vi "fgv_loop-dt_values.vi"() -> ()   [LabVIEW 2018]
panel:
  out "dt time arrays out":T1
  in  "dt time arrays":T1
  in  "cmd":enum16{"write", "read"}(ring)
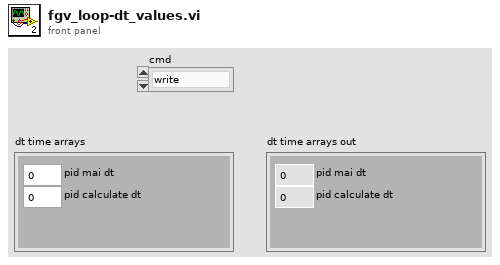
[diagram p1: front panel]
types:
  T1 = cluster{"pid mai dt":dbl, "pid calculate dt":dbl}
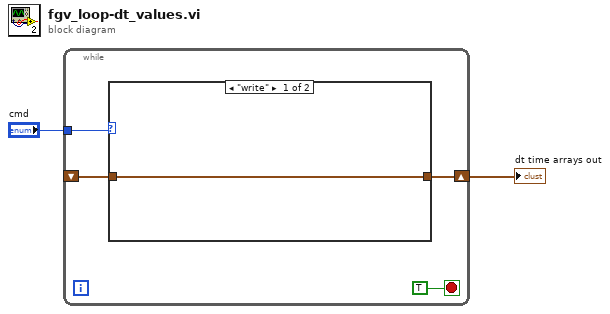
[diagram p0: block diagram]
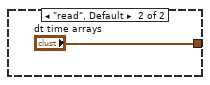
[diagram p2: hidden frame]
diagram:
  n1 = while {
    tunnel: "cmd" -> [w6]
    shift-right: [w4] -> w1
    shift-left: _ -> [w3]
    stop <- TRUE stop-if-true
    n2 = case shown="\"write\"" w6 {
      tunnel: [w7 "dt time arrays"] -> w4
      tunnel: w3 -> [w7 _]
      frame "write" {
      }
      frame "read", Default {
      }
    }
  }
  "dt time arrays out" <- w1
